vi "MotionProfileWriter.vi"(2 "startIndex":i32, 3 "ClearExistingMotionProfile":bool=TRUE, 4 "profileSlot1":i32, 5 "ProfileSlot0":i32, 6 "Trajectory Points":T6[](array[typedef]) {"Time (ms)" items=["TrajectoryDuration_0ms"=0, "TrajectoryDuration_5ms"=5, "TrajectoryDuration_10ms"=10, "TrajectoryDuration_20ms"=20, "TrajectoryDuration_30ms"=30, "TrajectoryDuration_40ms"=40, "TrajectoryDuration_50ms"=50, "TrajectoryDuration_100ms"=100]}, 7 "PhoenixMotorControlDevRef":T1={"DeviceStatus"={"status"=FALSE, "code"=0, "source"=""}, "Type"=enum."PWM", "PWM"={"PWM Channel"=enum."Invalid", "DeadBand"={"Name"="", "maxPositivePwm"=0, "minPositivePwm"=0, "centerPwm"=0, "maxNegativePwm"=0, "minNegativePwm"=0, "angularRange"=0}}, "CAN"={"Device Number"=0, "SetOutput VI Ref"=variant(enum8{"Percent VBus", "Current", "Speed", "Position", "Voltage"} enum."Percent VBus"), "GetOutput VI Ref"=variant(refnum<k1> refnum), "Enable VI Ref"=variant(dbl 12.0), "Disable VI Ref"=variant(enum8{"Percent VBus", "Speed", "Position", "Slave", "Unchanged / Invalid", "Voltage Compensation", "Current", "Motion Profile"} enum."Percent VBus"), "Data"=variant}, "Invert"=FALSE, "DIO PWM"={"PWM \"Enable\" Channel"=enum."Invalid", "DIOChannel"=enum."Invalid", "PWM Rate"=0.0}}) -> (0 "endIndex":i32, 1 "PhoenixMotorControlDevRef Out":T1={"DeviceStatus"={"status"=FALSE, "code"=0, "source"=""}, "Type"=enum."PWM", "PWM"={"PWM Channel"=enum."Invalid", "DeadBand"={"Name"="", "maxPositivePwm"=0, "minPositivePwm"=0, "centerPwm"=0, "maxNegativePwm"=0, "minNegativePwm"=0, "angularRange"=0}}, "CAN"={"Device Number"=0, "SetOutput VI Ref"=variant(enum8{"Percent VBus", "Current", "Speed", "Position", "Voltage"} enum."Percent VBus"), "GetOutput VI Ref"=variant(refnum<k1> refnum), "Enable VI Ref"=variant(dbl 12.0), "Disable VI Ref"=variant(enum8{"Percent VBus", "Speed", "Position", "Slave", "Unchanged / Invalid", "Voltage Compensation", "Current", "Motion Profile"} enum."Percent VBus"), "Data"=variant}, "Invert"=FALSE, "DIO PWM"={"PWM \"Enable\" Channel"=enum."Invalid", "DIOChannel"=enum."Invalid", "PWM Rate"=0.0}})   [LabVIEW 2017]
uses:
  TypeDefs/TrajectoryPoint.ctl
  <vilib>/Rock Robotics/WPI/ThirdParty/Phoenix-LabVIEW/Motor Controller/Controls/CTRE_Phoenix_MotorControl_TrajectoryPointTimeDur.ctl
  <vilib>/Rock Robotics/WPI/MotorControl/WPI_MotorControlDeviceRef.ctl
  <vilib>/Rock Robotics/WPI/MotorControl/WPI_MotorControlType.ctl
  <vilib>/Rock Robotics/SystemInterfaces/DIO/FPGA_DIOPWMChannel.ctl
  <vilib>/Rock Robotics/WPI/PWM/WPI_PWMDeadband.ctl
  <vilib>/Rock Robotics/SystemInterfaces/DIO/FPGA_DIOChannel.ctl
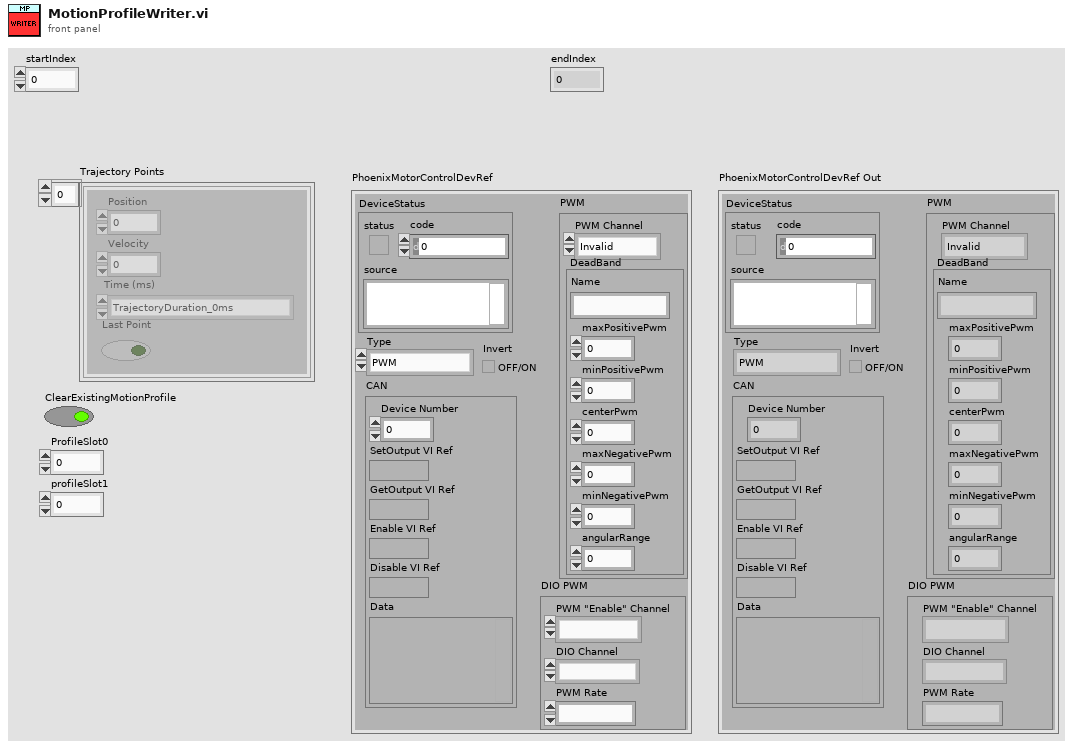
[diagram p1: front panel]
types:
  T1 = typedef "WPI_MotorControlDeviceRef.ctl" = cluster{"DeviceStatus":errorcluster, "Type":T2, "PWM":cluster{"PWM Channel":T3, "DeadBand":T4}, "CAN":cluster{"Device Number":u8, "SetOutput VI Ref":variant, "GetOutput VI Ref":variant, "Enable VI Ref":variant, "Disable VI Ref":variant, "Data":variant}, "Invert":bool, "DIO PWM":cluster{"PWM \"Enable\" Channel":T3, "DIOChannel":T5, "PWM Rate":dbl}}
  T2 = typedef "WPI_MotorControlType.ctl" = enum16{"PWM", "CAN", "DIO PWM"}
  T3 = typedef "FPGA_DIOPWMChannel.ctl" = enum8{"PWM 0", "PWM 1", "PWM 2", "PWM 3", "PWM 4", "PWM 5", "PWM 6", "PWM 7", "PWM 8", "PWM 9", "PWM MXP 0", "PWM MXP 1", "PWM MXP 2", "PWM MXP 3", "PWM MXP 4", "PWM MXP 5", "PWM MXP 6", "PWM MXP 7", "PWM MXP 8", "PWM MXP 9", "Invalid"}
  T4 = typedef "WPI_PWMDeadband.ctl" = cluster{"Name":string, "maxPositivePwm":i32, "minPositivePwm":i32, "centerPwm":i32, "maxNegativePwm":i32, "minNegativePwm":i32, "angularRange":u16}
  T5 = typedef "FPGA_DIOChannel.ctl" = enum8{"DIO 0", "DIO 1", "DIO 2", "DIO 3", "DIO 4", "DIO 5", "DIO 6", "DIO 7", "DIO 8", "DIO 9", "DIO MXP 0", "DIO MXP 1", "DIO MXP 2", "DIO MXP 3", "DIO MXP 4", "DIO MXP 5", "DIO MXP 6", "DIO MXP 7", "DIO MXP 8", "DIO MXP 9", "DIO MXP 10", "DIO MXP 11", "DIO MXP 12", "DIO MXP 13", "DIO MXP 14", "DIO MXP 15", "SPI Port CS1", "SPI Port CS2", "SPI Port CS3", "SPI Port MISO", "SPI Port MOSI", "Invalid"}
  T6 = typedef "TrajectoryPoint.ctl" = cluster{"Position ":dbl, "Velocity ":dbl, "Time (ms)":T7, "Last Point":bool}
  T7 = typedef "CTRE_Phoenix_MotorControl_TrajectoryPointTimeDur.ctl" = i32
  T8 = cluster{"Top Buffer Remaining":i32, "Top Buffer Count":i32, "Bottom Buffer Count":i32, "Has Underrun?":bool, "Is Underrun?":bool, "Active Point Valid?":bool, "Is Last?":bool, "Profile Slot Select 0":i32, "Output Enable":i32, "Time Duration (ms)":i32, "Profile Slot Select 1":i32}
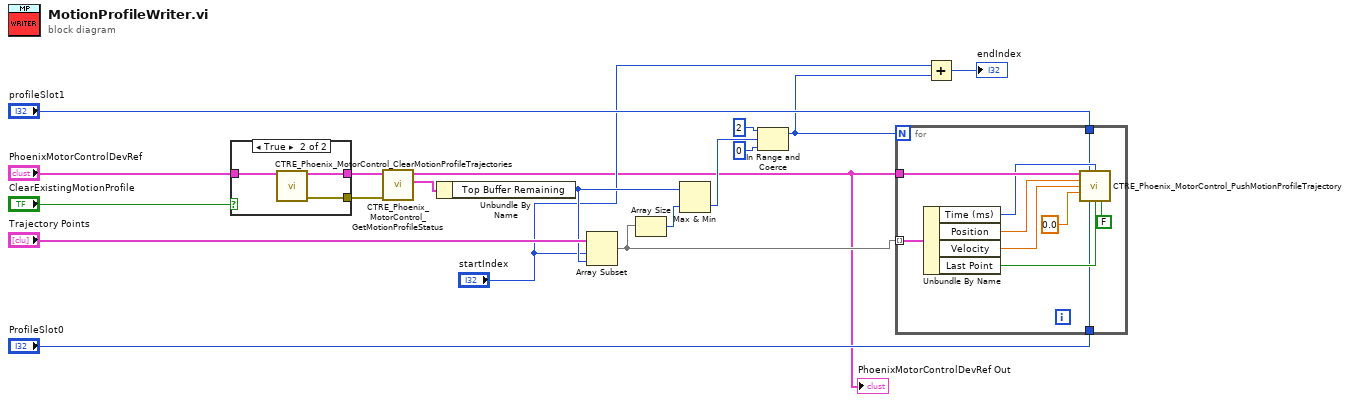
[diagram p0: block diagram]
diagram:
  n1 = case shown="True" "ClearExistingMotionProfile" {
    tunnel: "PhoenixMotorControlDevRef" -> [w19 w22]
    tunnel: [w19 w21] -> w14
    tunnel: [_ w20] -> w12
    frame False {
    }
    frame True {
      n2 = call <vilib>:"CTRE_Phoenix_MotorControl_ClearMotionProfileTrajectories.vi"("PhoenixMotorControlDevRef"=w22) -> ("PhoenixMotorControlDevRef"=w21:T1, "error out"=w20:errorcluster)  [unwired: 13 in]
    }
  }
  n3 = call <vilib>:"CTRE_Phoenix_MotorControl_GetMotionProfileStatus.vi"("error in"=w12, "PhoenixMotorControlDevRef"=w14) -> ("Motion Profile Status"=w13:T8, "PhoenixMotorControlDevRef"=w1:T1)  [unwired: 7 in, 1 out]
  "PhoenixMotorControlDevRef Out" <- w1
  n4 = Unbundle By Name(w13) -> ("Top Buffer Remaining"=w8:i32)
  n5 = Array Subset(array="Trajectory Points", index="startIndex", length=w8) -> (w10:T6[])
  n6 = Array Size(array=w10) -> (size(s)=w9:i32)
  n7 = Max & Min(x=w8, y=w9) -> (min(x,y)=w3:i32)  [unwired: 1 out]
  n8 = In Range and Coerce(upper limit=2 ("x"), x=w3, lower limit=0) -> (coerced(x)=w4:i32)  [unwired: 1 out]
  n9 = for {
    N: w4 -> [_]
    tunnel: "ProfileSlot0" -> [w24]
    tunnel: w1 -> [w32]
    tunnel: w10 -> [w31] mode=indexing
    tunnel: "profileSlot1" -> [w23]
    n10 = Unbundle By Name(w31) -> ("Time (ms)"=w27:T7, "Position"=w30:dbl, "Velocity"=w29:dbl, "Last Point"=w28:bool)
    n11 = call <vilib>:"CTRE_Phoenix_MotorControl_PushMotionProfileTrajectory.vi"("PhoenixMotorControlDevRef"=w32, "profileSlotSelect1"=w23, "durationMs"=w27, "position"=w30, "velocity"=w29, "headingDeg"=0.0, "profileSlotSelect0"=w24, "isLastPoint?"=w28, "Zero Position?"=FALSE) -> ()  [unwired: 5 in, 2 out]
  }
  n12 = Add(x="startIndex", y=w4) -> (x+y=→"endIndex":i32)
